vi "EnabletChannelVI.vi"(0 "Angelsample":dbl[](array[numeric]), 1 "Angel":bool[](array[boolean]), 2 "dt":dbl, 5 "Torquesample":dbl[](array[numeric]), 7 "Torque":bool[](array[boolean]), 9 "ResetAngel":dbl[](array[numeric]), 11 "ResetTorqueCommand":dbl[](array[numeric]), 12 "ChannelSetArray":T1[](array[typedef]) {"Enable" items=["不使能", "使能"]; "Wave" items=["0指令", "正弦波", "方波", "三角波", "常值", "波形数据", "白噪声", "正弦扫频", "梯度加载", "VMIC"]; "ChannelType" items=["标准波形跟踪"=1, "扫频测试"=2, "消除多余力"=3, "梯度加载"=4, "载荷谱跟踪"=5, "模拟输入跟踪"=9]; "ChannelStatus" items=["通道关", "位置通道", "加载通道"]}, 13 "AxisForceSample":dbl[](array[numeric])) -> (4 "ControlOutput":dbl[](array[numeric]), 6 "resetAngel 2":dbl[](array[numeric]), 10 "ResetTorque 2":dbl[](array[numeric]), 15 "Commandout":dbl[](array[numeric]))   [LabVIEW 2020]
uses:
  ChannelCommand.ctl
  Control 1.ctl
  WaveType.ctl
  MoterEnable.ctl
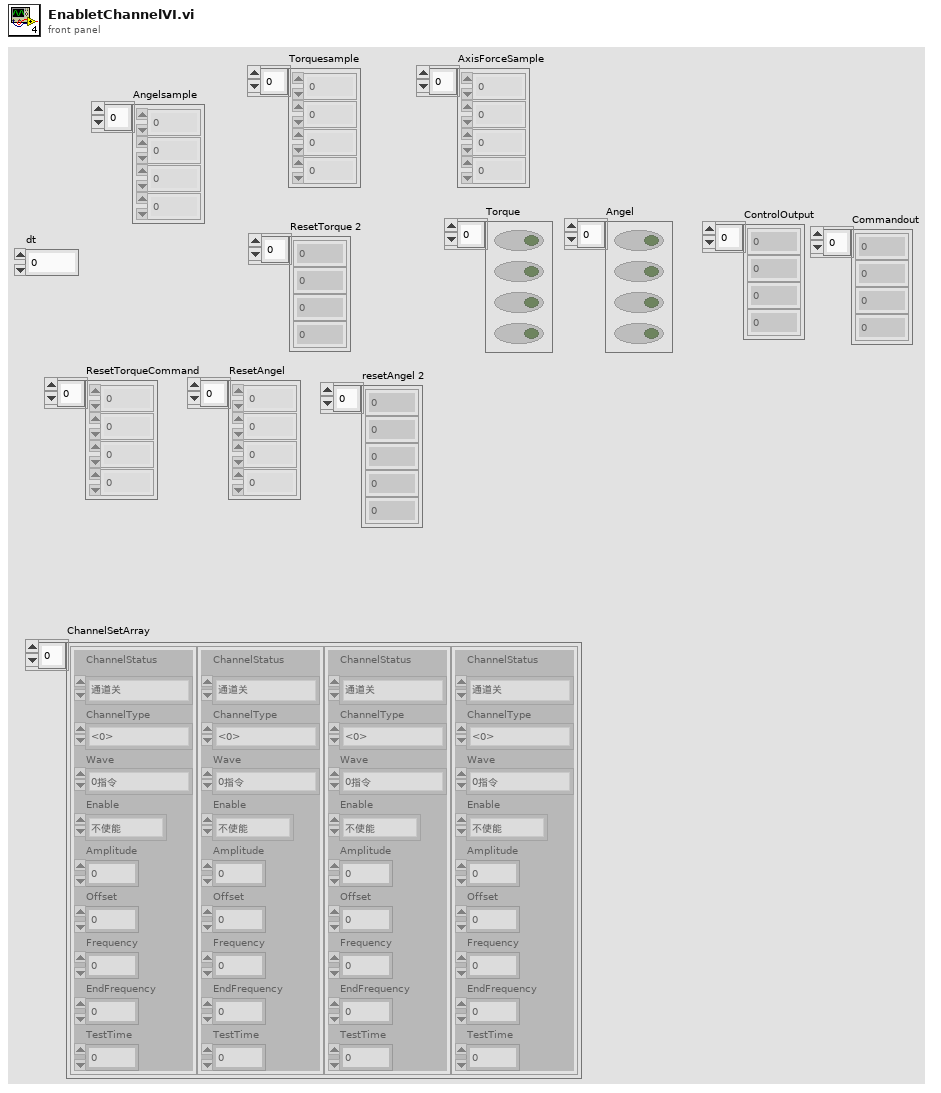
[diagram p1: front panel]
types:
  T1 = typedef "ChannelCommand.ctl" = cluster{"ChannelStatus":T2, "ChannelType":i32, "Wave":T3, "Enable":T4, "Amplitude":dbl, "Offset":dbl, "Frequency":dbl, "EndFrequency":dbl, "TestTime":dbl}
  T2 = typedef "Control 1.ctl" = i32
  T3 = typedef "WaveType.ctl" = i32
  T4 = typedef "MoterEnable.ctl" = u16
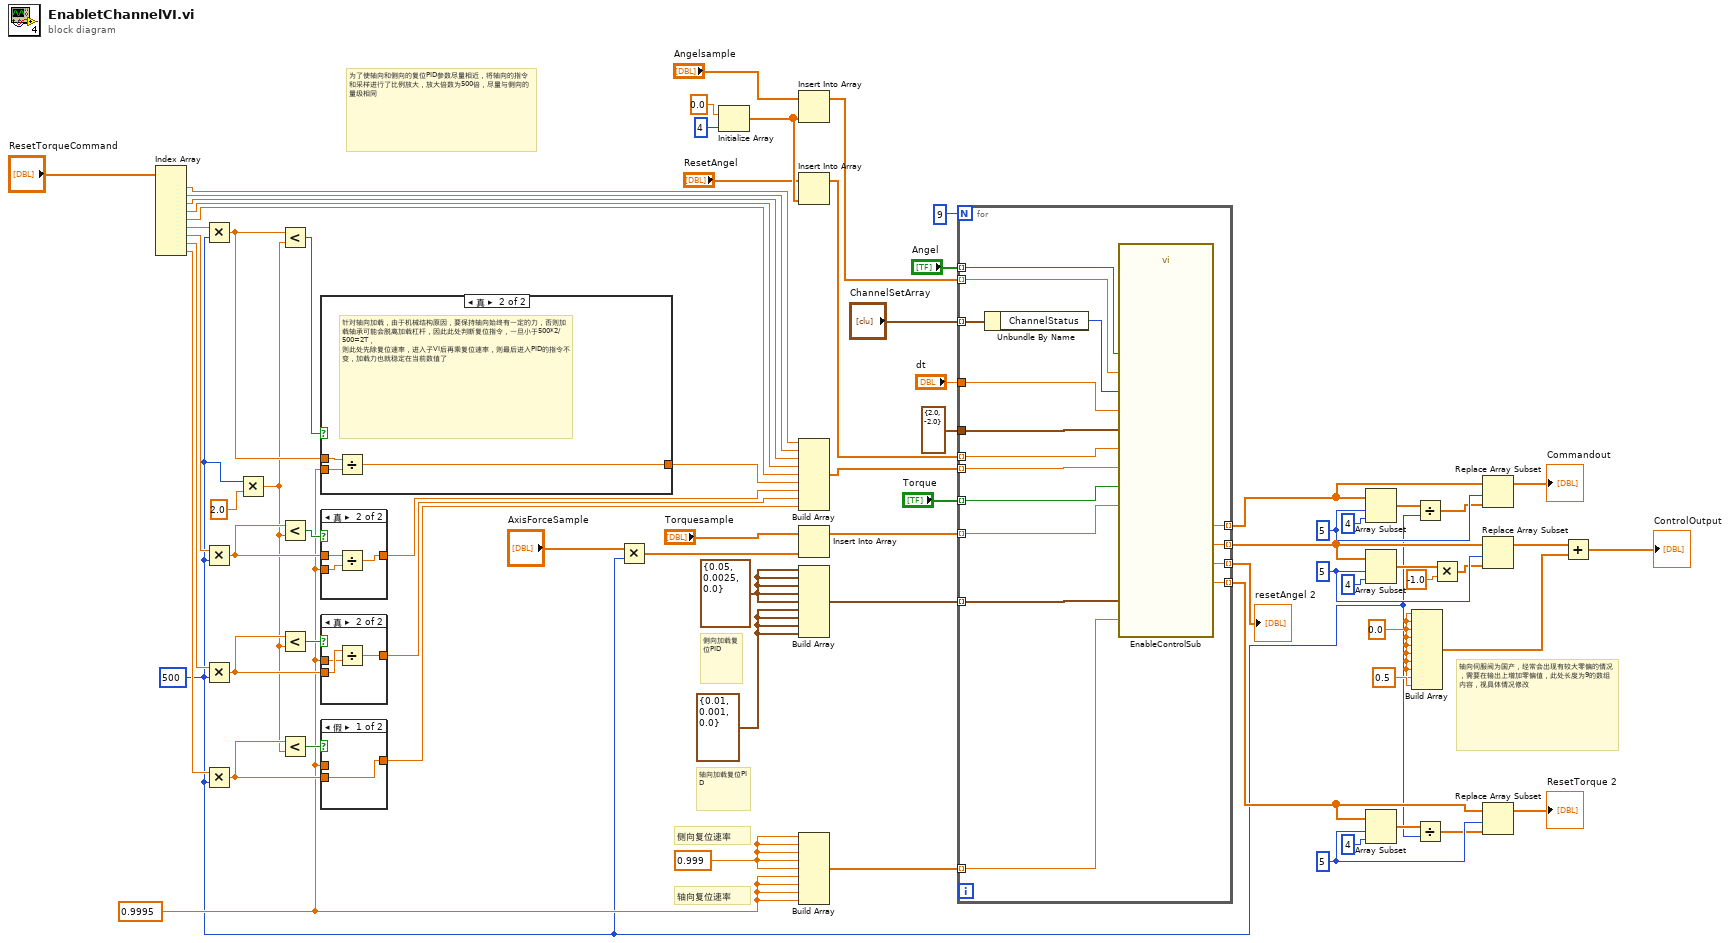
[diagram p0: block diagram]
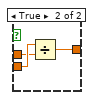
[diagram p2: hidden frame]
diagram:
  w5 = 0.0
  w15 = 5 ("索引")
  w21 = 5 ("索引")
  w26 = 5 ("索引")
  w4 = 0.9995
  w54 = 0.999
  w57 = cluster{dbl, dbl, dbl} {0.05, 0.0025, 0.0} ("簇")
  w56 = cluster{dbl, dbl, dbl} {0.01, 0.001, 0.0} ("簇")
  w2 = 500
  # "为了使轴向和侧向的复位PID参数尽量相近，将轴向的指令和采样进行了比例放大，放大倍数为500倍，尽量与侧向的量级相同"
  # "轴向伺服阀为国产，经常会出现有较大零偏的情况，需要在输出上增加零偏值，此处长度为9的数组内容，视具体情况修改"
  # "轴向复位速率"
  # "侧向复位速率"
  # "轴向加载复位PID"
  # "侧向加载复位PID"
  n1 = Index Array(array="ResetTorqueCommand") -> (element #1=w38:dbl, element #2=w37:dbl, element #3=w36:dbl, element #4=w35:dbl, element #5=w34:dbl, element #6=w39:dbl, element #7=w40:dbl, element #8=w41:dbl, element #9=w42:dbl)  [unwired: 9 in]
  n2 = Multiply(x=w39, y=w2) -> (x*y=w70:dbl)
  n3 = Multiply(x=w40, y=w2) -> (x*y=w66:dbl)
  n4 = Multiply(x=w41, y=w2) -> (x*y=w65:dbl)
  n5 = Multiply(x=w42, y=w2) -> (x*y=w64:dbl)
  n6 = Multiply(x=w2, y=2.0) -> (x*y=w1:dbl)
  n7 = Less?(x=w70, y=w1) -> (x < y?=w71:bool)
  n8 = Less?(x=w66, y=w1) -> (x < y?=w69:bool)
  n9 = Less?(x=w65, y=w1) -> (x < y?=w68:bool)
  n10 = Less?(x=w64, y=w1) -> (x < y?=w67:bool)
  n11 = case shown="真" w71 {
    tunnel: w70 -> [w74 w77]
    tunnel: [w74 w76] -> w33
    tunnel: w4 -> [_ w75]
    frame False {
    }
    frame True {
      # "针对轴向加载，由于机械结构原因，要保持轴向始终有一定的力，否则加载轴承可能会脱离加载杠杆，因此此处判断复位指令，一旦小于500*2/500=2T，\n则此处先除复位速率，进入子VI后再乘复位速率，则最后进入PID的指令不变，加载力也就稳定在当前数值了"
      n12 = Divide(x=w77, y=w75) -> (x/y=w76:dbl)
    }
  }
  n13 = case shown="真" w69 {
    tunnel: w66 -> [w78 w81]
    tunnel: [w78 w80] -> w32
    tunnel: w4 -> [_ w79]
    frame False {
    }
    frame True {
      n14 = Divide(x=w81, y=w79) -> (x/y=w80:dbl)
    }
  }
  n15 = case shown="真" w68 {
    tunnel: w65 -> [w82 w85]
    tunnel: [w82 w84] -> w31
    tunnel: w4 -> [_ w83]
    frame False {
    }
    frame True {
      n16 = Divide(x=w85, y=w83) -> (x/y=w84:dbl)
    }
  }
  n17 = case shown="假" w67 {
    tunnel: w64 -> [w86 w89]
    tunnel: [w86 w88] -> w30
    tunnel: w4 -> [_ w87]
    frame False {
    }
    frame True {
      n18 = Divide(x=w89, y=w87) -> (x/y=w88:dbl)
    }
  }
  n19 = Multiply(x="AxisForceSample", y=w2) -> (x*y=w51:dbl[])
  n20 = Initialize Array(0.0 ("元素"), 4 ("维数大小")) -> (w45:dbl[])
  n21 = Insert Into Array(array="Angelsample", new element=w45) -> (w46:dbl[])  [unwired: 1 in]
  n22 = Insert Into Array(array="ResetAngel", new element=w45) -> (w43:dbl[])  [unwired: 1 in]
  n23 = Build Array(w38, w37, w36, w35, w34, w33, w32, w31, w30) -> (w29:dbl[])
  n24 = Insert Into Array(array="Torquesample", new element=w51) -> (w50:dbl[])  [unwired: 1 in]
  n25 = Build Array(w57, w57, w57, w57, w57, w56, w56, w56, w56) -> (w55:cluster{dbl, dbl, dbl}[])
  n26 = Build Array(w54, w54, w54, w54, w54, w4, w4, w4, w4) -> (w53:dbl[])
  n27 = for {
    N: 9 -> [_]
    tunnel: "Angel" -> [w105] mode=indexing
    tunnel: "Torque" -> [w104] mode=indexing
    tunnel: "ChannelSetArray" -> [w103] mode=indexing
    tunnel: "dt" -> [w101]
    tunnel: cluster{"output high":dbl, "output low":dbl} {"output high"=2.0, "output low"=-2.0} ("output range") -> [w100]
    tunnel: w55 -> [w99] mode=indexing
    tunnel: w53 -> [w98] mode=indexing
    tunnel: w50 -> [w97] mode=indexing
    tunnel: w46 -> [w96] mode=indexing
    tunnel: w43 -> [w95] mode=indexing
    tunnel: w29 -> [w94] mode=indexing
    tunnel: [w93] -> w27 mode=indexing
    tunnel: [w92] -> w18 mode=indexing
    tunnel: [w91] -> w10 mode=indexing
    tunnel: [w90] -> w14 mode=indexing
    n28 = Unbundle By Name(w103) -> ("ChannelStatus"=w102:T2)
    n29 = call "EnableControlSub.vi"("dt"=w101, "Torque"=w104, "ResetAngle"=w95, "复位速率"=w98, "TorqueSample"=w97, "Angel"=w105, "AngleSample"=w96, "ChannelStatus"=w102, "ResetTorque"=w94, "output range"=w100, "ResetPID"=w99) -> ("ResetTorque 2"=w92:dbl, "ResetAngle 2"=w91:dbl, "ControlOutput"=w90:dbl, "Commandout"=w93:dbl)  [unwired: 1 in]
  }
  "resetAngel 2" <- w10
  n30 = Array Subset(array=w27, index=w26, length=4 ("长度")) -> (w25:dbl[])
  n31 = Array Subset(array=w14, index=w15, length=4 ("长度")) -> (w13:dbl[])
  n32 = Array Subset(array=w18, index=w21, length=4 ("长度")) -> (w20:dbl[])
  n33 = Build Array(w5, w5, w5, w5, w5, w5, w5, w5, w5, 0.5) -> (w8:dbl[])
  n34 = Divide(x=w25, y=w2) -> (x/y=w24:dbl[])
  n35 = Divide(x=w20, y=w2) -> (x/y=w19:dbl[])
  n36 = Multiply(x=w13, y=-1.0) -> (x*y=w12:dbl[])
  n37 = Replace Array Subset(array=w27, new element=w24, index=w26) -> (→"Commandout":dbl[])
  n38 = Replace Array Subset(array=w14, new element=w12, index=w15) -> (w7:dbl[])
  n39 = Replace Array Subset(array=w18, new element=w19, index=w21) -> (→"ResetTorque 2":dbl[])
  n40 = Add(x=w7, y=w8) -> (x+y=→"ControlOutput":dbl[])
